vi "UnitTest-SizeAsRoot.vi"(8 "error in":errorcluster) -> (0 "error out":errorcluster)   [LabVIEW 2014]
uses:
  TableLogger_Actor/TableLoggerConfig.ctl
  TableLogger_Actor/TableLoggerTypes.ctl
  TableLogger_Actor/TableLoggerBackupConfig.ctl
  <vilib>/addons/_JKI Toolkits/Caraya/classes/Assert/Assert.lvclass
  <vilib>/addons/_JKI Toolkits/Caraya/classes/Test/Test.lvclass
  TableLogger_Actor/TableLogger_Actor.lvlib
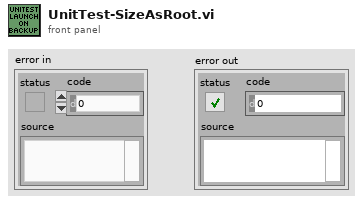
[diagram p1: front panel]
types:
  T1 = typedef "TableLogger_Actor.lvlib/TableLoggerConfig.ctl" = cluster{"TableLogger":T2, "DB File Path":path, "DB Backup Config":T3}
  T2 = typedef "TableLogger_Actor.lvlib/TableLoggerTypes.ctl" = enum16{"CSV Logger", "SQLite Logger"}
  T3 = typedef "TableLogger_Actor.lvlib/TableLoggerBackupConfig.ctl" = cluster{"Directory":path, "UTC Time Format":bool, "On Launch":bool, "Interval (Hours)":dbl, "Size Multiples (Bytes)":i32}
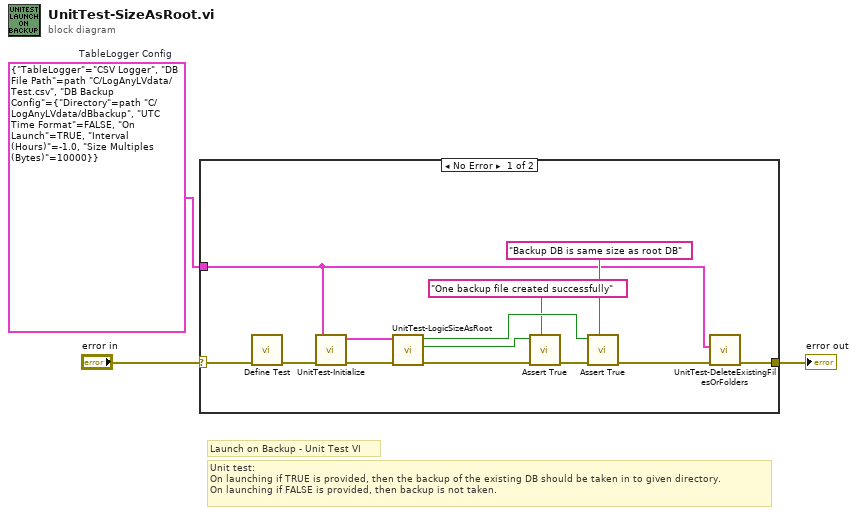
[diagram p0: block diagram]
diagram:
  w3 = T1 {"TableLogger"=enum."CSV Logger", "DB File Path"=path "C:/LogAnyLVdata/Test.csv", "DB Backup Config"={"Directory"=path "C:/LogAnyLVdata/dBbackup", "UTC Time Format"=FALSE, "On Launch"=TRUE, "Interval (Hours)"=-1.0, "Size Multiples (Bytes)"=10000}}  # TableLogger Config
  # "Unit test:\nOn launching if TRUE is provided, then the backup of the existing DB should be taken in to given directory.\nOn launching if FALSE is provided, then backup is not taken."
  # "Launch on Backup - Unit Test VI"
  n1 = case shown="No Error" "error in" {
    selector: "error in" -> [w16 w17]
    tunnel: w3 -> [w4 _]
    tunnel: [w11 w17] -> w2
    frame No Error {
      n2 = call <vilib>:"Define Test.vi"("error in (no error)"=w16) -> ("error out"=w7:errorcluster)  [unwired: 10 in]
      n3 = call "UnitTest-Initialize.vi"("error in"=w7, "Config IN"=w4) -> ("error out"=w6:errorcluster, "Config OUT"=w5:T1)  [unwired: 7 in, 1 out]
      n4 = call "UnitTest-LogicSizeAsRoot.vi"("error in (no error)"=w6, ">> Config >>"=w5) -> ("error out"=w9:errorcluster, "Dir?T"=w13:bool, "DataSize?Equal"=w14:bool)  [unwired: 7 in]
      n5 = call <vilib>:"Assert True.vi"("Label"="One backup file created successfully", "error in (no error)"=w9, "True?"=w13) -> ("error out"=w10:errorcluster)  [unwired: 8 in]
      n6 = call <vilib>:"Assert True.vi"("Label"="Backup DB is same size as root DB", "error in (no error)"=w10, "True?"=w14) -> ("error out"=w8:errorcluster)  [unwired: 8 in]
      n7 = call "UnitTest-DeleteExistingFilesOrFolders.vi"("error in (no error)"=w8, "Config IN"=w4) -> ("error out"=w11:errorcluster)  [unwired: 9 in]
    }
    frame Error {
    }
  }
  "error out" <- w2
